vi "Wordle Results.vi"() -> ()   [LabVIEW 2020]
uses:
  <vilib>/drjdpowell/SQLite Library/SQL Statement/SQL Statement.lvclass/SQL Statement.ctl
  User Score.ctl
  SoL Scoring/Score.ctl
  SoL Scoring/Score Entry.ctl
  <vilib>/Utility/miscctls.llb/LVMapReplaceAction.ctl
  <vilib>/drjdpowell/SQLite Library/SQL Statement/Column I64.vi
  89ce5cd6-0151-4ce3-a17e-ba547d2c57c4.vi
  e7392ecc-94d6-418e-9175-70b81eeff3ff.vi
  931bc3dd-bffb-44c4-bbc3-12f1a34549e5.vi
  2a2c68d8-e587-4431-8f6d-11a2ebca744d.vi
  0f526391-7734-4541-91be-b0151a8a595a.vi
  2b5a74f5-1657-4fea-9533-5163be9a7f4a.vi
  <vilib>/drjdpowell/SQLite Library/SQL Statement/Bind Integer.vi
  <vilib>/drjdpowell/SQLite Library/SQL Statement/Error Message.vi
  <vilib>/drjdpowell/SQLite Library/SQL Statement/Column String.vi
  <vilib>/Comparison/Less/Less Functor/Less Functor.lvclass
  SQLite/SQLite.lvclass
  <vilib>/drjdpowell/SQLite Library/SQL Connection/Connection.lvclass
  <vilib>/drjdpowell/SQLite Library/SQL Statement/SQL Statement.lvclass
  SoL Scoring/SoL Scoring.lvlib
  Summer of LabVIEW.lvlib
panel:
  in  "DB File":path
  in  "Submissions":path
  out "Smallest LLB":T1(array[cluster])
  out "Fewest Most Guesses":T1(array[cluster])
  out "Count":T1(array[cluster])
  out "Fastest":T1(array[cluster])
  out "Score":T1(array[cluster])
  out "Most Improved":T1(array[cluster])
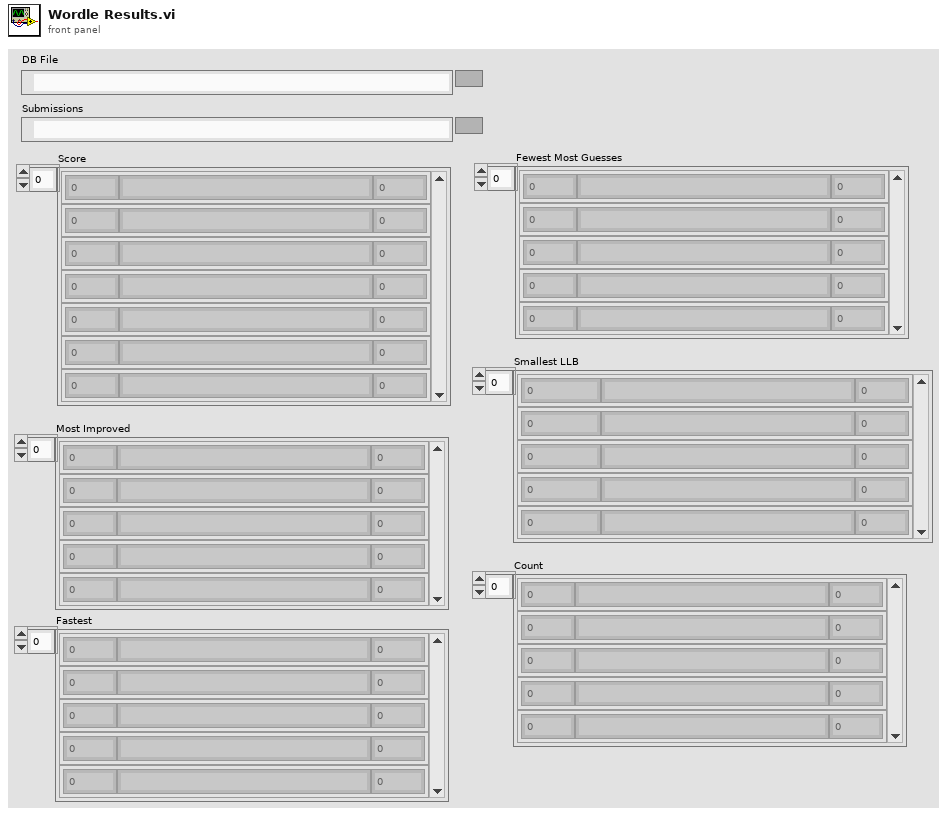
[diagram p1: front panel]
types:
  T1 = cluster{dbl, "Submitter":string, "user_id":i64}[]
  T2 = map{i64, cluster{"Most Guesses Required":dbl, "Least Guesses Required":dbl, "Total Solve Time":dbl, "Score":dbl, "Submitter":string, "user_id":i64, "sub_id":i64}[]}
  T3 = cluster{"Most Guesses Required":dbl, "Least Guesses Required":dbl, "Total Solve Time":dbl, "Score":dbl, "Submitter":string, "user_id":i64, "sub_id":i64}
  T4 = typedef "SoL Scoring.lvlib/Score.ctl" = cluster{"Overall":dbl, "Categories":T5[]}
  T5 = typedef "SoL Scoring.lvlib/Score Entry.ctl" = cluster{"Category":string, "Value":dbl}
  T6 = typedef "Summer of LabVIEW.lvlib/User Score.ctl" = cluster{"first_name":string, "last_name":string, "department":string, "score":T4, "user_id":i64, "sub_id":i64, "chal_id":i64}
  T7 = typedef "LVMapReplaceAction.ctl" = enum32{"Modify Entry only if found", "Add or Modify Entry", "Delete Entry"}
  T8 = cluster{"Most Guesses Required":dbl, "Least Guesses Required":dbl, "Total Solve Time":dbl, "Score":dbl, "Submitter":string, "user_id":i64, "sub_id":i64}[]
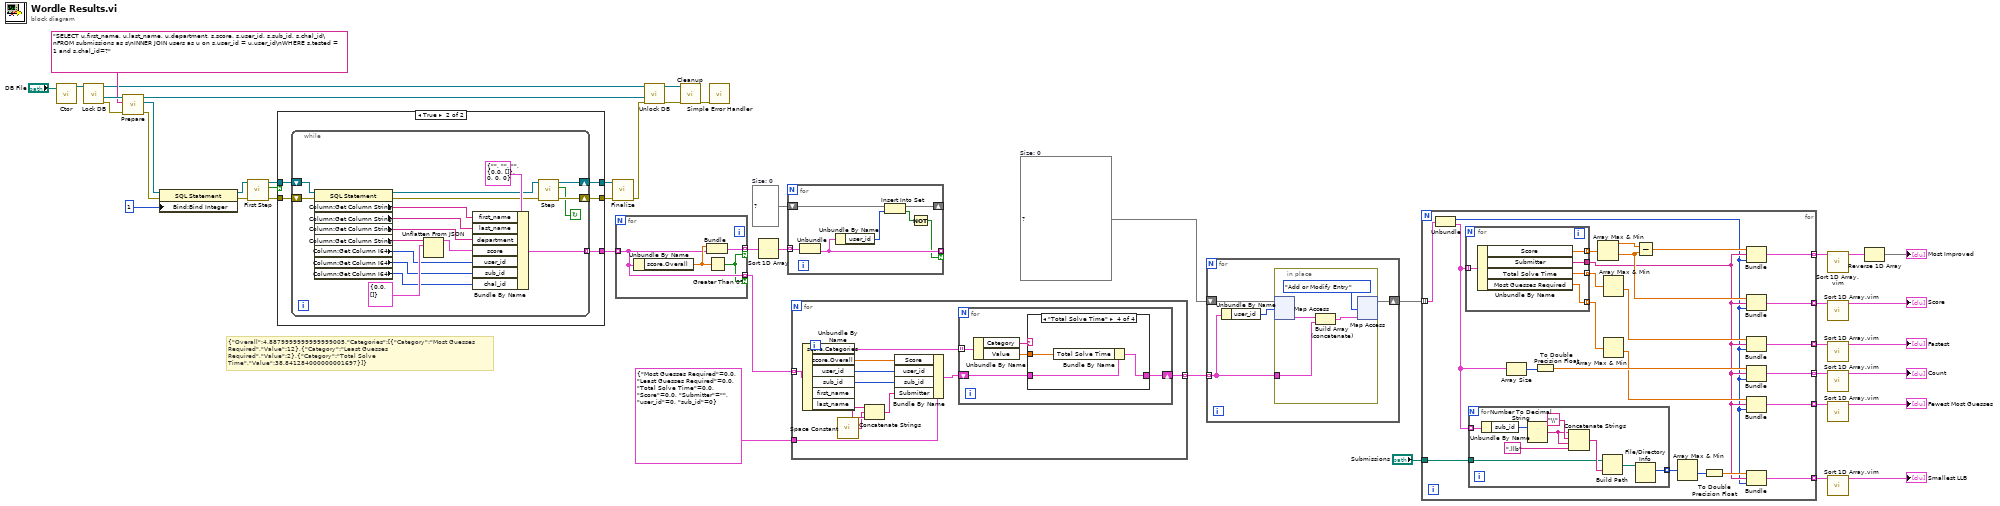
[diagram p0: block diagram]
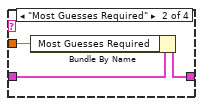
[diagram p3: hidden frame]
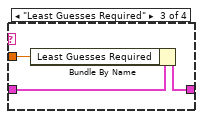
[diagram p4: hidden frame]
diagram:
  w19 = T2 {}  # Size: 0
  w26 = set{i64} {}  # Size: 0
  # "{\"Overall\":4.8879999999999999005,\"Categories\":[{\"Category\":\"Most Guesses Required\",\"Value\":12},{\"Category\":\"Least Guesses Required\",\"Value\":2},{\"Category\":\"Total Solve Time\",\"Value\":38.841284000000001697}]}"
  n1 = call "Ctor.vi"("DB File"="DB File") -> ("SQLite out"=w24:refnum<class "SQLite.lvclass">)  [unwired: 9 in, 1 out]
  n2 = call "Lock DB.vi"("SQLite in"=w24) -> ("error out"=w41:errorcluster, "SQLite DB"=w44:refnum<class "Connection.lvclass">, "SQLite out"=w32:refnum<class "SQLite.lvclass">)  [unwired: 7 in, 1 out]
  n3 = call <vilib>:"Prepare.vi"("error in (no error)"=w41, "SQL"="SELECT u.first_name, u.last_name, u.department, s.score, s.user_id, s.sub_id, s.chal_id\nFROM submissions as s\nINNER JOIN users as u on s.user_id = u.user_id\nWHERE s.tested = 1 and s.chal_id=?", "SQLite Connection in"=w44) -> ("error out"=w40:errorcluster, "SQL Statement"=w42:refnum<class "SQL Statement.lvclass">, "SQLite Connection"=w30:refnum<class "Connection.lvclass">)  [unwired: 4 in, 2 out]
  n4 = property class="SQL Statement"(reference=w42, error in=w40, "Bind:Bind Integer"=i64 1 ("Challenge ID")) -> (reference out=w39:refnum<class "SQL Statement.lvclass">, error out=w38:errorcluster)
  n5 = call <vilib>:"First Step.vi"("error in (no error)"=w38, "SQL Statement in"=w39) -> ("error out"=w35:errorcluster, "Row returned"=w37:bool, "SQL Statement"=w36:refnum<class "SQL Statement.lvclass">)  [unwired: 7 in]
  n6 = case shown="True" w37 {
    tunnel: w36 -> [w46 w51]
    tunnel: w35 -> [w45 w50]
    tunnel: [w46 w49] -> w33
    tunnel: [w45 w48] -> w34
    tunnel: [_ w47] -> w29
    frame False {
    }
    frame True {
      n7 = while {
        shift-right: [w54] -> w49
        shift-left: w51 -> [w69]
        tunnel: [w57] -> w47 mode=indexing
        shift-right: [w53] -> w48
        shift-left: w50 -> [w68]
        stop <- w52 continue-if-true
        n8 = property class="SQL Statement"(reference=w69, error in=w68) -> (reference out=w55:refnum<class "SQL Statement.lvclass">, error out=w56:errorcluster, "Column:Get Column String"=w66:string, "Column:Get Column String"=w65:string, "Column:Get Column String"=w64:string, "Column:Get Column String"=w63:string, "Column:Get Column I64"=w60:i64, "Column:Get Column I64"=w59:i64, "Column:Get Column I64"=w58:i64)
        n9 = Unflatten From JSON(JSON string=w63, type and defaults=T4 {"Overall"=0.0, "Categories"=[]} ("Score")) -> (value=w61:T4)  [unwired: 5 in, 1 out]
        n10 = Bundle By Name(cluster=T6 {"first_name"="", "last_name"="", "department"="", "score"={"Overall"=0.0, "Categories"=[]}, "user_id"=0, "sub_id"=0, "chal_id"=0} ("User Score"), "first_name"=w66, "last_name"=w65, "department"=w64, "score"=w61, "user_id"=w60, "sub_id"=w59, "chal_id"=w58) -> (w57:T6)
        n11 = call <vilib>:"Step.vi"("error in (no error)"=w56, "SQL Statement in"=w55) -> ("error out"=w53:errorcluster, "Row returned"=w52:bool, "SQL Statement"=w54:refnum<class "SQL Statement.lvclass">)  [unwired: 7 in]
      }
    }
  }
  n12 = call <vilib>:"Finalize.vi"("error in (no error)"=w34, "SQL Statement in"=w33) -> ("error out"=w31:errorcluster)  [unwired: 9 in]
  n13 = for {
    tunnel: w29 -> [w71] mode=indexing
    tunnel: [w73] -> w28 mode=indexing if=w70
    tunnel: [w71] -> w21 mode=indexing if=w70
    n14 = Unbundle By Name(w71) -> ("score.Overall"=w72:dbl)
    n15 = Bundle("Overall"=w72, "User Score"=w71) -> (w73:cluster{"Overall":dbl, "User Score":T6})  [unwired: 1 in]
    n16 = Greater Than 0?(x=w72) -> (x > 0?=w70:bool)
  }
  n17 = call "Unlock DB.vi"("error in (no error)"=w31, "SQLite DB"=w30, "SQLite in"=w32) -> ("error out"=w22:errorcluster, "SQLite out"=w23:refnum<class "SQLite.lvclass">)  [unwired: 7 in]
  n18 = call-dynamic "Cleanup.vi"("error in (no error)"=w22, "SQLite in"=w23) -> ("error out"=w3:errorcluster)  [unwired: 9 in]
  n19 = call <vilib>:"Simple Error Handler.vi"("error in (no error)"=w3) -> ()  [unwired: 4 in, 5 out]
  n20 = Sort 1D Array(array=w28) -> (sorted array=w27:cluster{"Overall":dbl, "User Score":T6}[])
  n21 = for {
    tunnel: w27 -> [w80] mode=indexing
    tunnel: [w79] -> _ mode=indexing if=w74
    shift-right: [w75] -> _
    shift-left: w26 -> [w78]
    n22 = Unbundle(w80) -> ("User Score"=w79:T6)  [unwired: 1 out]
    n23 = Unbundle By Name(w79) -> ("user_id"=w77:i64)
    n24 = Insert Into Set(10:w77, 11:w78) -> (2:w76:bool, 3:w75:set{i64})
    n25 = Not(x=w76) -> (.not. x?=w74:bool)
  }
  n26 = for {
    tunnel: w21 -> [w91] mode=indexing
    tunnel: T3 {"Most Guesses Required"=0.0, "Least Guesses Required"=0.0, "Total Solve Time"=0.0, "Score"=0.0, "Submitter"="", "user_id"=0, "sub_id"=0} -> [w92]
    tunnel: [w87] -> w18 mode=indexing
    n27 = Unbundle By Name(w91) -> ("score.Categories"=w89:T5[], "score.Overall"=w90:dbl, "user_id"=w82:i64, "sub_id"=w81:i64, "first_name"=w86:string, "last_name"=w85:string)
    n28 = call <vilib>:"Space Constant.vi"() -> ("String"=w84:string)
    n29 = Concatenate Strings(w86, w84, w85) -> (w83:string)
    n30 = Bundle By Name(cluster=w92, "Score"=w90, "user_id"=w82, "sub_id"=w81, "Submitter"=w83) -> (w88:T3)
    n31 = for {
      tunnel: w89 -> [w97] mode=indexing
      shift-right: [w93] -> w87
      shift-left: w88 -> [w94]
      n32 = Unbundle By Name(w97) -> ("Category"=w96:string, "Value"=w95:dbl)
      n33 = case shown="\"Total Solve Time\"" w96 {
        tunnel: w95 -> [_ w100 w103 w106]
        tunnel: w94 -> [w98 w101 w104 w107]
        tunnel: [w98 w99 w102 w105] -> w93
        frame Default {
        }
        frame "Most Guesses Required" {
          n34 = Bundle By Name(cluster=w101, "Most Guesses Required"=w100) -> (w99:T3)
        }
        frame "Least Guesses Required" {
          n35 = Bundle By Name(cluster=w104, "Least Guesses Required"=w103) -> (w102:T3)
        }
        frame "Total Solve Time" {
          n36 = Bundle By Name(cluster=w107, "Total Solve Time"=w106) -> (w105:T3)
        }
      }
    }
  }
  n37 = for {
    shift-right: [w108] -> w17
    shift-left: w19 -> [w111]
    tunnel: w18 -> [w109] mode=indexing
    n38 = Unbundle By Name(w109) -> ("user_id"=w110:i64)
    n39 = in-place {
      in-place-border: w109 -> [w114]
      n40 = in-place-map #1(w111, w110) -> (w115:T8)  [unwired: 1 in, 1 out]
      n41 = Build Array (concatenate)(w115, w114) -> (w113:T8)
      n42 = in-place-map #1(w113, LVMapReplaceAction."Add or Modify Entry" ("action")) -> (w108:T2)  [unwired: 2 out]
    }
  }
  n43 = for {
    tunnel: w17 -> [w139] mode=indexing
    tunnel: [w135] -> w16 mode=indexing
    tunnel: [w133] -> w13 mode=indexing
    tunnel: [w130] -> w11 mode=indexing
    tunnel: [w128] -> w8 mode=indexing
    tunnel: [w125] -> w7 mode=indexing
    tunnel: "Submissions" -> [w122]
    tunnel: [w116] -> w4 mode=indexing
    n44 = Unbundle(w139) -> ("user_id"=w117:i64, w123:T8)
    n45 = for {
      tunnel: w123 -> [w144] mode=indexing
      tunnel: [w143] -> w138 mode=indexing
      tunnel: [w142] -> w118
      tunnel: [w141] -> w132 mode=indexing
      tunnel: [w140] -> w126 mode=indexing
      n46 = Unbundle By Name(w144) -> ("Score"=w143:dbl, "Submitter"=w142:string, "Total Solve Time"=w141:dbl, "Most Guesses Required"=w140:dbl)
    }
    n47 = for {
      tunnel: w123 -> [w153] mode=indexing
      tunnel: w122 -> [w147]
      tunnel: [w145] -> w121 mode=indexing
      n48 = Unbundle By Name(w153) -> ("sub_id"=w152:i64)
      n49 = Number To Decimal String(number=w152) -> (decimal integer string=w150:string)  [unwired: 1 in]
      n50 = Concatenate Strings(w150, "\\" ("string"), w150, ".llb" ("string")) -> (w148:string)
      n51 = Build Path(base path=w147, name or relative path=w148) -> (appended path=w146:path)
      n52 = File/Directory Info(path=w146) -> (size=w145:i64)  [unwired: 1 in, 6 out]
    }
    n53 = Array Size(array=w123) -> (size(s)=w129:i32)
    n54 = To Double Precision Float(number=w129) -> (double precision float=w127:dbl)
    n55 = Array Max & Min(array=w138) -> (max value=w137:dbl, min value=w134:dbl)  [unwired: 2 out]
    n56 = Array Max & Min(array=w132) -> (min value=w131:dbl)  [unwired: 3 out]
    n57 = Array Max & Min(array=w126) -> (min value=w124:dbl)  [unwired: 3 out]
    n58 = Subtract(x=w137, y=w134) -> (x-y=w136:dbl)
    n59 = Array Max & Min(array=w121) -> (min value=w120:i64)  [unwired: 3 out]
    n60 = To Double Precision Float(number=w120) -> (double precision float=w119:dbl)
    n61 = Bundle(w136, "Submitter"=w118, "user_id"=w117) -> (w135:cluster{dbl, "Submitter":string, "user_id":i64})  [unwired: 1 in]
    n62 = Bundle(w134, "Submitter"=w118, "user_id"=w117) -> (w133:cluster{dbl, "Submitter":string, "user_id":i64})  [unwired: 1 in]
    n63 = Bundle(w131, "Submitter"=w118, "user_id"=w117) -> (w130:cluster{dbl, "Submitter":string, "user_id":i64})  [unwired: 1 in]
    n64 = Bundle(w127, "Submitter"=w118, "user_id"=w117) -> (w128:cluster{dbl, "Submitter":string, "user_id":i64})  [unwired: 1 in]
    n65 = Bundle(w124, "Submitter"=w118, "user_id"=w117) -> (w125:cluster{dbl, "Submitter":string, "user_id":i64})  [unwired: 1 in]
    n66 = Bundle(w119, "Submitter"=w118, "user_id"=w117) -> (w116:cluster{dbl, "Submitter":string, "user_id":i64})  [unwired: 1 in]
  }
  n67 = call "Sort 1D Array.vim"("unsorted array"=w16) -> ("sorted array"=w15:T1)  [unwired: 10 in]
  n68 = call "Sort 1D Array.vim"("unsorted array"=w13) -> ("sorted array"=→"Score":T1)  [unwired: 10 in]
  n69 = call "Sort 1D Array.vim"("unsorted array"=w11) -> ("sorted array"=→"Fastest":T1)  [unwired: 10 in]
  n70 = call "Sort 1D Array.vim"("unsorted array"=w8) -> ("sorted array"=→"Count":T1)  [unwired: 10 in]
  n71 = call "Sort 1D Array.vim"("unsorted array"=w7) -> ("sorted array"=→"Fewest Most Guesses":T1)  [unwired: 10 in]
  n72 = call "Sort 1D Array.vim"("unsorted array"=w4) -> ("sorted array"=→"Smallest LLB":T1)  [unwired: 10 in]
  n73 = Reverse 1D Array(array=w15) -> (reversed array=→"Most Improved":T1)
